vi "CreateWriteMessage.vi"(2 "Value":i32, 3 "Address":u32, 4 "Device":u8=1) -> (1 "Message":string)   [LabVIEW 2021]
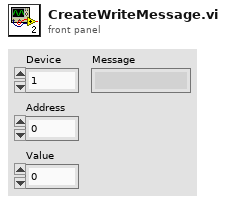
[diagram p1: front panel]
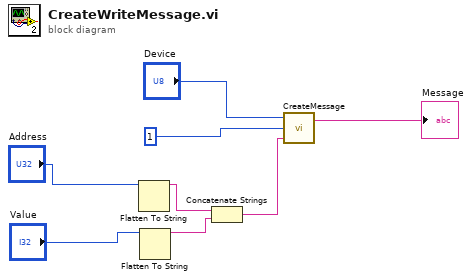
[diagram p0: block diagram]
diagram:
  n1 = Flatten To String(anything="Address") -> (data string=w6:string)  [unwired: 3 in, 2 out]
  n2 = Flatten To String(anything="Value") -> (data string=w5:string)  [unwired: 3 in, 2 out]
  n3 = Concatenate Strings(w6, w5) -> (w4:string)
  n4 = call "CreateMessage.vi"("Payload"=w4, "Operation"=u8 1, "Device"="Device") -> ("Message"=→"Message":string)  [unwired: 1 in]
